vi "modulo.vi"() -> ()   [LabVIEW 2014]
panel:
  out "a % b":dbl
  in  "b":dbl
  in  "a":dbl
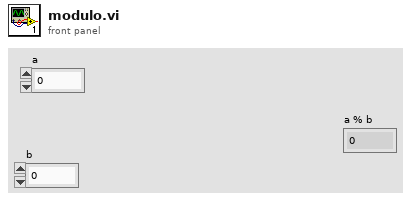
[diagram p1: front panel]
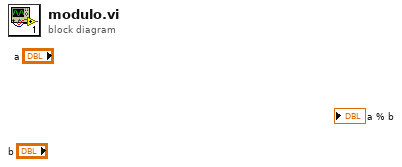
[diagram p0: block diagram]
diagram:
